vi "PH_Cam_BaseClass.Setting Packer.vi"(3 "error in (no error)":errorcluster, 5 "Cam Settings In":T1={"Cam ID"="N/A", "Gain"=nan, "Brightness"=nan, "Shutter"=nan, "Mode"=-1}) -> (0 "error out":errorcluster, 1 "Cam Settings":string[](array[string]), 2 "Cam Settings Out":T1={"Cam ID"="N/A", "Gain"=nan, "Brightness"=nan, "Shutter"=nan, "Mode"=-1})   [LabVIEW 2014, in "PH_Cam_BaseClass.lvlib"]
doc: "This VI labels the cam settings and packs them to a string array."
uses:
  PH_Cam_BaseClass.lvlib
  PH_Cam_BaseClass.Settings.ctl
  PH_Common/PH_Common.lvlib
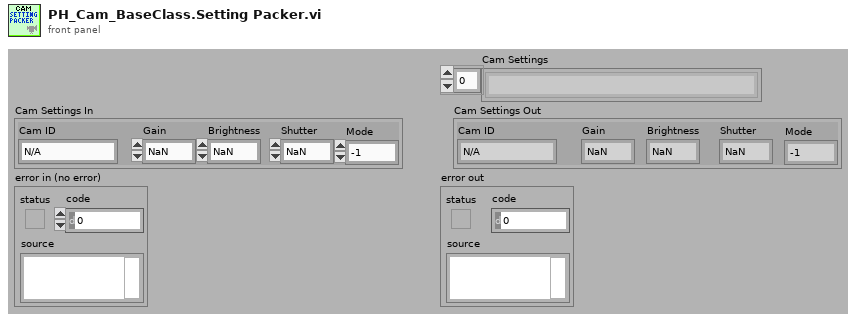
[diagram p1: front panel]
types:
  T1 = typedef "PH_Cam_BaseClass.lvlib/PH_Cam_BaseClass.Settings.ctl" = cluster{"Cam ID":string, "Gain":dbl, "Brightness":dbl, "Shutter":dbl, "Mode":i32}
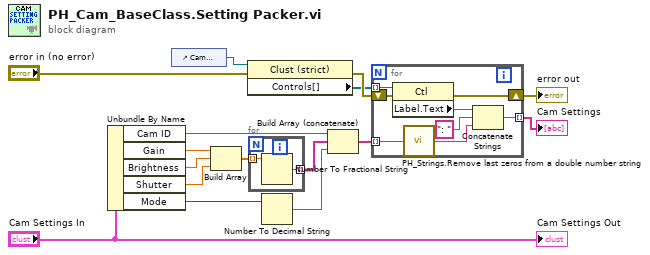
[diagram p0: block diagram]
diagram:
  n1 = Unbundle By Name("Cam Settings In") -> ("Cam ID"=w13:string, "Gain"=w12:dbl, "Brightness"=w11:dbl, "Shutter"=w10:dbl, "Mode"=w3:i32)
  n2 = control-ref of="Cam Settings In"() -> (w1:refnum<vi>)
  n3 = Build Array(w12, w11, w10) -> (w7:dbl[])
  n4 = property class="Clust (strict)"(reference=w1, error in="error in (no error)") -> (error out=w15:errorcluster, "Controls[]"=w14:refnum<vi>[])  [unwired: 1 out]
  n5 = for {
    tunnel: w7 -> [w17] mode=indexing
    tunnel: [w18] -> w6 mode=indexing
    n6 = Number To Fractional String(number=w17) -> (F-format string=w18:string)  [unwired: 3 in]
  }
  n7 = Number To Decimal String(number=w3) -> (decimal integer string=w2:string)  [unwired: 1 in]
  n8 = Build Array (concatenate)(w13, w6, w2) -> (w8:string[])
  n9 = for {
    tunnel: w14 -> [w26] mode=indexing
    shift-right: [w24] -> w16
    shift-left: w15 -> [w25]
    tunnel: [w21] -> w9 mode=indexing
    tunnel: w8 -> [w20] mode=indexing
    n10 = property class="Ctl"(reference=w26, error in=w25) -> (error out=w24:errorcluster, "Label.Text"=w22:string)  [unwired: 1 out]
    n11 = call "PH_Strings.Remove last zeros from a double number string.vi"("String in"=w20) -> ("String out"=w19:string)
    n12 = Concatenate Strings(w22, ": " ("string"), w19) -> (w21:string)
  }
  "error out" <- w16
  "Cam Settings" <- w9
  "Cam Settings Out" <- "Cam Settings In"
